vi "Util_Trajectory_WriteFile_Config.vi"(9 "TRAJECTORY_CONFIG":T1 {"End Velocity" format="%20.4f"; "StartVelocity" format="%20.4f"; "Max Acceleration" format="%20.4f"; "MaxVelocity" format="%20.4f"}, 11 "Byte Steam File In":refnum<file>) -> (0 "error out":errorcluster, 3 "Byte Steam File Out":refnum<file>)   [LabVIEW 2019, in "Trajectory_Library.lvlib"]
doc: "Internal routine to write the Trajectory Configuration data to a file.\n\nParameters:\n - ByteStream In - File stream\n - TrajectoryConfig - Data structure containing trajectory configuration\n\nReturns:\n - ByteStream Out - File stream\n - Error out - returned error cluster\n\nReturns:\n - outTrajectory - Trajectory data structure\n - Error out - returned error cluster"
uses:
  Trajectory_Library.lvlib
  TypeDef/TRAJ_CONFIG.ctl
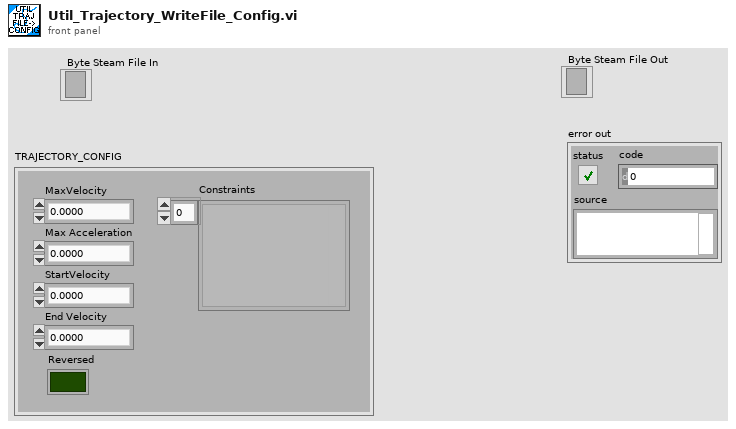
[diagram p1: front panel]
types:
  T1 = typedef "Trajectory_Library.lvlib/TRAJ_CONFIG.ctl" = cluster{"MaxVelocity":dbl, "Max Acceleration":dbl, "StartVelocity":dbl, "End Velocity":dbl, "Reversed":bool, "Constraints":variant[]}
  T2 = typedef "WPILib_Math.lvlib/TRAJ_CONSTRAINT_DIIF_DRIVE_KINEMATICS.ctl" = cluster{"Max Speed (M/S)":dbl, "DIFF_DRIVE_KINEMATICS":T3, "Max Accel (M/S2)":dbl}
  T3 = typedef "WPILib_Math.lvlib/DIFF_DRIVE_KINEMATICS.ctl" = cluster{"TrackWidth_Meters":dbl}
  T4 = typedef "Trajectory_Library.lvlib/TRAJ_CONSTRAINT_DIIF_DRIVE_VOLTAGE.ctl" = cluster{"Max Voltage":dbl, "DIFF_DRIVE_KINEMATICS":T5, "SIMPLE_MOTOR_FF":T6}
  T5 = typedef "Trajectory_Library.lvlib/DIFF_DRIVE_KINEMATICS.ctl" = cluster{"TrackWidth_Meters":dbl}
  T6 = typedef "Trajectory_Library.lvlib/SIMPLE_MOTOR_FF.ctl" = cluster{"Ks":dbl, "Kv":dbl, "Ka":dbl, "KnInv":dbl}
  T7 = typedef "Trajectory_Library.lvlib/TRAJ_CONSTRAINT_SWERVE_DRIVE_KINEMATICS.ctl" = cluster{"Max Speed (M/S)":dbl, "SwerveKinematics":T8}
  T8 = typedef "Trajectory_Library.lvlib/SWERVE_DRIVE_KINEMATICS.ctl" = cluster{"NumModules":i32, "InverseKinematics":T9, "ForwardKinematics":T9, "Modules":T10[], "PrevCoR":T10, "SavedModuleStates":T11[]}
  T9 = typedef "NI_Matrix.lvlib/RealMatrix.ctl" = dbl[][]
  T10 = typedef "Trajectory_Library.lvlib/TRANSLATION2D.ctl" = cluster{"X":dbl, "Y":dbl}
  T11 = typedef "Trajectory_Library.lvlib/SWERVE_DRIVE_MODULE_STATE.ctl" = cluster{"Speed":dbl, "Angle":T12}
  T12 = typedef "Trajectory_Library.lvlib/ROTATION2D.ctl" = cluster{"VALUE":dbl, "COS":dbl, "SIN":dbl}
  T13 = typedef "Trajectory_Library.lvlib/TRAJ_CONSTRAINT_MECA_DRIVE_KINEMATICS.ctl" = cluster{"Max Speed (M/S)":dbl, "MECA_DRIVE_KINEMATICS":T14}
  T14 = typedef "Trajectory_Library.lvlib/MECA_DRIVE_KINEMATICS.ctl" = cluster{"FrontLeft":T10, "FrontRight":T10, "RearLeft":T10, "RearRight":T10, "InverseKinematics":T9, "ForwardKinematics":T9, "PrevCoR":T10}
  T15 = typedef "Trajectory_Library.lvlib/TRAJ_CONSTRAINT_CENTRIPETAL_ACCEL.ctl" = cluster{"Max Cent Accel":dbl}
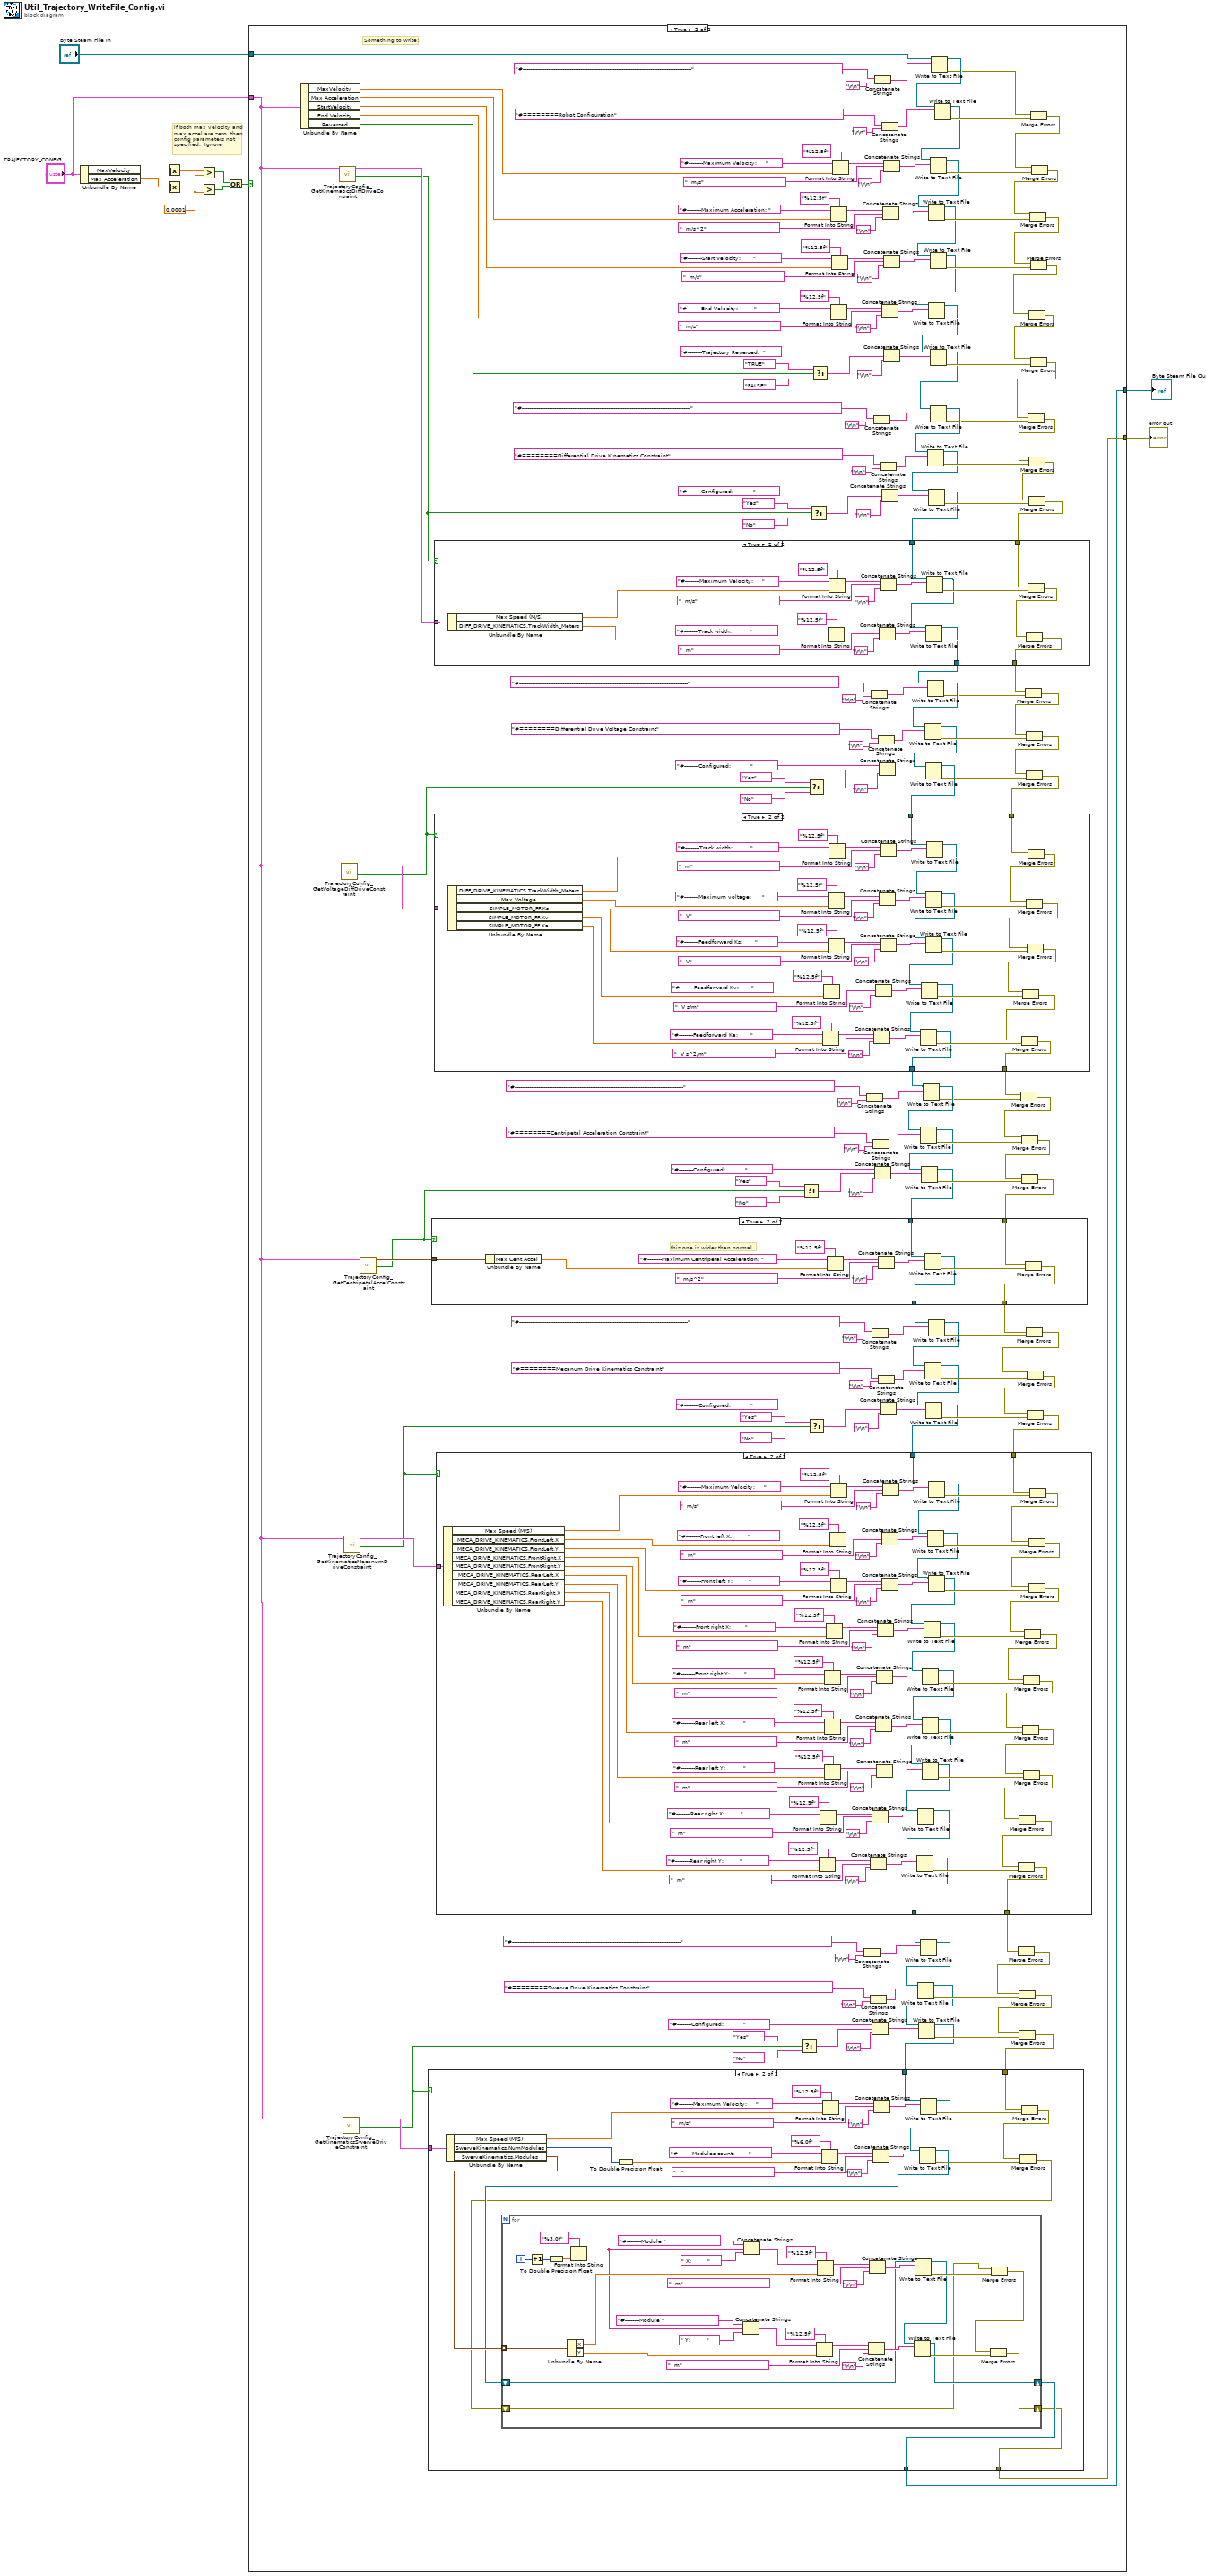
[diagram p0: block diagram]
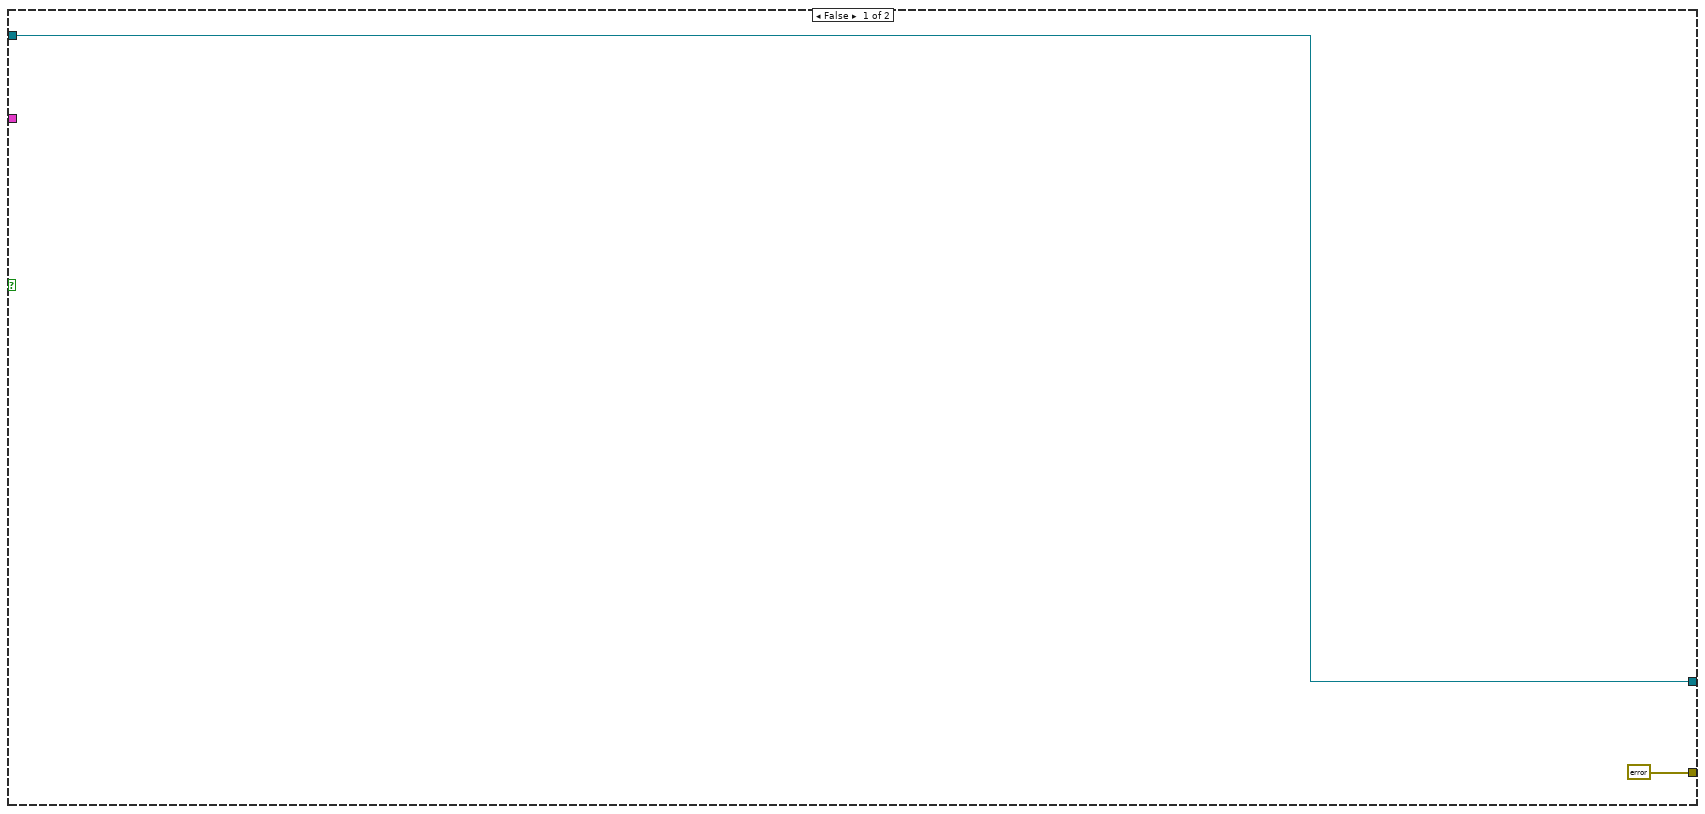
[diagram p2: hidden frame]
diagram:
  w5 = 0.0001
  # "if both max velocity and\nmax accel are zero, then\nconfig parameters not\nspecified.  Ignore"
  n1 = Unbundle By Name("TRAJECTORY_CONFIG") -> ("MaxVelocity"=w8:dbl, "Max Acceleration"=w9:dbl)
  n2 = Absolute Value(x=w8) -> (abs(x)=w7:dbl)
  n3 = Absolute Value(x=w9) -> (abs(x)=w6:dbl)
  n4 = Greater?(x=w7, y=w5) -> (0:w4:bool)
  n5 = Greater?(x=w6, y=w5) -> (0:w3:bool)
  n6 = Or(x=w4, y=w3) -> (x .or. y?=w2:bool)
  n7 = case shown="True" w2 {
    tunnel: [w14 w26] -> w12
    tunnel: "Byte Steam File In" -> [w14 w196]
    tunnel: [errorcluster {"status"=FALSE, "code"=0, "source"=""} ("error out") w27] -> w10
    tunnel: "TRAJECTORY_CONFIG" -> [_ w15]
    frame False {
    }
    frame True {
      # "Something to write!"
      n8 = Unbundle By Name(w15) -> ("MaxVelocity"=w182:dbl, "Max Acceleration"=w181:dbl, "StartVelocity"=w163:dbl, "End Velocity"=w162:dbl, "Reversed"=w161:bool)
      n9 = call "TrajectoryConfig_GetKinematicsDiffDriveContraint.vi"("inTRAJECTORY_CONFIG"=w15) -> ("Constraint Exists"=w24:bool, "Diff Drive Kinematics Constraint"=w25:T2)  [unwired: 9 in]
      n10 = call "TrajectoryConfig_GetVoltageDiffDriveConstraint.vi"("inTRAJECTORY_CONFIG"=w15) -> ("Constraint Exists"=w22:bool, "Differential Drive Voltage Constraint"=w23:T4)  [unwired: 9 in]
      n11 = call "TrajectoryConfig_GetKinematicsSwerveDriveConstraint.vi"("inTRAJECTORY_CONFIG"=w15) -> ("Constraint Exists"=w16:bool, "Swerver Drive Kinematics Constraint"=w19:T7)  [unwired: 9 in]
      n12 = call "TrajectoryConfig_GetKinematicsMecanumDriveConstraint.vi"("inTRAJECTORY_CONFIG"=w15) -> ("Constraint Exists"=w17:bool, "Mecanum Drive Kinematics Constraint"=w18:T13)  [unwired: 9 in]
      n13 = call "TrajectoryConfig_GetCentripetalAccelConstraint.vi"("inTRAJECTORY_CONFIG"=w15) -> ("Constraint Exists"=w20:bool, "Centripital Accleration Constraint"=w21:T15)  [unwired: 9 in]
      n14 = Select(t="Yes" ("string"), s=w16, f="No" ("string")) -> (s? t:f=w79:string)
      n15 = Select(t="Yes" ("string"), s=w20, f="No" ("string")) -> (s? t:f=w111:string)
      n16 = Select(t="Yes" ("string"), s=w22, f="No" ("string")) -> (s? t:f=w127:string)
      n17 = Select(t="Yes" ("string"), s=w17, f="No" ("string")) -> (s? t:f=w95:string)
      n18 = Select(t="Yes" ("string"), s=w24, f="No" ("string")) -> (s? t:f=w151:string)
      n19 = Select(t="TRUE" ("string"), s=w161, f="FALSE" ("string")) -> (s? t:f=w167:string)
      n20 = Format Into String(format string="%12.5f", initial string="#--------End Velocity:         " ("string"), w162) -> (resulting string=w171:string)  [unwired: 1 in, 1 out]
      n21 = Format Into String(format string="%12.5f", initial string="#--------Maximum Acceleration: " ("string"), w181) -> (resulting string=w183:string)  [unwired: 1 in, 1 out]
      n22 = Format Into String(format string="%12.5f", initial string="#--------Start Velocity:       " ("string"), w163) -> (resulting string=w176:string)  [unwired: 1 in, 1 out]
      n23 = Format Into String(format string="%12.5f", initial string="#--------Maximum Velocity:     " ("string"), w182) -> (resulting string=w188:string)  [unwired: 1 in, 1 out]
      n24 = Concatenate Strings("#----------------------------------------------------------------------------------------------" ("string"), "\r\n") -> (w83:string)
      n25 = Concatenate Strings("#----------------------------------------------------------------------------------------------" ("string"), "\r\n") -> (w115:string)
      n26 = Concatenate Strings("#========Swerve Drive Kinematics Constraint" ("string"), "\r\n") -> (w86:string)
      n27 = Concatenate Strings("#----------------------------------------------------------------------------------------------" ("string"), "\r\n") -> (w131:string)
      n28 = Concatenate Strings("#----------------------------------------------------------------------------------------------" ("string"), "\r\n") -> (w99:string)
      n29 = Concatenate Strings("#--------Configured:           " ("string"), w79, "\r\n") -> (w81:string)
      n30 = Concatenate Strings("#========Centripetal Acceleration Constraint" ("string"), "\r\n") -> (w118:string)
      n31 = Concatenate Strings("#----------------------------------------------------------------------------------------------" ("string"), "\r\n") -> (w155:string)
      n32 = Concatenate Strings("#----------------------------------------------------------------------------------------------" ("string"), "\r\n") -> (w197:string)
      n33 = Concatenate Strings("#--------Configured:           " ("string"), w111, "\r\n") -> (w113:string)
      n34 = Concatenate Strings("#========Differential Drive Voltage Constraint" ("string"), "\r\n") -> (w134:string)
      n35 = Concatenate Strings("#========Mecanum Drive Kinematics Constraint" ("string"), "\r\n") -> (w102:string)
      n36 = Concatenate Strings("#--------Configured:           " ("string"), w127, "\r\n") -> (w129:string)
      n37 = Concatenate Strings("#--------Configured:           " ("string"), w95, "\r\n") -> (w97:string)
      n38 = Concatenate Strings("#========Differential Drive Kinematics Constraint" ("string"), "\r\n") -> (w158:string)
      n39 = Concatenate Strings("#========Robot Configuration" ("string"), "\r\n") -> (w200:string)
      n40 = Concatenate Strings(w171, "  m/s" ("string"), "\r\n") -> (w173:string)
      n41 = Concatenate Strings("#--------Configured:           " ("string"), w151, "\r\n") -> (w153:string)
      n42 = Concatenate Strings(w183, "  m/s^2" ("string"), "\r\n") -> (w185:string)
      n43 = Concatenate Strings(w176, "  m/s" ("string"), "\r\n") -> (w178:string)
      n44 = Concatenate Strings("#--------Trajectory Reversed:  " ("string"), w167, "\r\n") -> (w169:string)
      n45 = Concatenate Strings(w188, "  m/s" ("string"), "\r\n") -> (w192:string)
      n46 = Write to Text File(file (use dialog)=w196, text=w197) -> (refnum out=w195:refnum<file>, error out=w189:errorcluster)  [unwired: 2 in, 1 out]
      n47 = Write to Text File(file (use dialog)=w195, text=w200) -> (refnum out=w72:refnum<file>, error out=w191:errorcluster)  [unwired: 2 in, 1 out]
      n48 = Write to Text File(file (use dialog)=w72, text=w192) -> (refnum out=w71:refnum<file>, error out=w190:errorcluster)  [unwired: 2 in, 1 out]
      n49 = Write to Text File(file (use dialog)=w71, text=w185) -> (refnum out=w70:refnum<file>, error out=w184:errorcluster)  [unwired: 2 in, 1 out]
      n50 = Write to Text File(file (use dialog)=w70, text=w178) -> (refnum out=w69:refnum<file>, error out=w177:errorcluster)  [unwired: 2 in, 1 out]
      n51 = Write to Text File(file (use dialog)=w69, text=w173) -> (refnum out=w68:refnum<file>, error out=w172:errorcluster)  [unwired: 2 in, 1 out]
      n52 = Write to Text File(file (use dialog)=w68, text=w169) -> (refnum out=w67:refnum<file>, error out=w168:errorcluster)  [unwired: 2 in, 1 out]
      n53 = Write to Text File(file (use dialog)=w67, text=w155) -> (refnum out=w147:refnum<file>, error out=w137:errorcluster)  [unwired: 2 in, 1 out]
      n54 = Write to Text File(file (use dialog)=w147, text=w158) -> (refnum out=w66:refnum<file>, error out=w138:errorcluster)  [unwired: 2 in, 1 out]
      n55 = Write to Text File(file (use dialog)=w66, text=w153) -> (refnum out=w65:refnum<file>, error out=w152:errorcluster)  [unwired: 2 in, 1 out]
      n56 = Merge Errors(w189, w191) -> (w55:errorcluster)
      n57 = Merge Errors(w55, w190) -> (w54:errorcluster)
      n58 = Merge Errors(w54, w184) -> (w53:errorcluster)
      n59 = Merge Errors(w53, w177) -> (w52:errorcluster)
      n60 = Merge Errors(w52, w172) -> (w51:errorcluster)
      n61 = Merge Errors(w51, w168) -> (w50:errorcluster)
      n62 = Merge Errors(w50, w137) -> (w49:errorcluster)
      n63 = Merge Errors(w49, w138) -> (w48:errorcluster)
      n64 = Merge Errors(w48, w152) -> (w47:errorcluster)
      n65 = case shown="True" w24 {
        tunnel: w25 -> [_ w453]
        tunnel: w65 -> [w430 w436]
        tunnel: [w430 w434] -> w64
        tunnel: w47 -> [w429 w433]
        tunnel: [w429 w431] -> w46
        frame False {
        }
        frame True {
          n66 = Unbundle By Name(w453) -> ("Max Speed (M/S)"=w442:dbl, "DIFF_DRIVE_KINEMATICS.TrackWidth_Meters"=w441:dbl)
          n67 = Format Into String(format string="%12.5f", initial string="#--------Track width:          " ("string"), w441) -> (resulting string=w443:string)  [unwired: 1 in, 1 out]
          n68 = Format Into String(format string="%12.5f", initial string="#--------Maximum Velocity:     " ("string"), w442) -> (resulting string=w448:string)  [unwired: 1 in, 1 out]
          n69 = Concatenate Strings(w443, "  m" ("string"), "\r\n") -> (w445:string)
          n70 = Concatenate Strings(w448, "  m/s" ("string"), "\r\n") -> (w450:string)
          n71 = Write to Text File(file (use dialog)=w436, text=w450) -> (refnum out=w435:refnum<file>, error out=w449:errorcluster)  [unwired: 2 in, 1 out]
          n72 = Write to Text File(file (use dialog)=w435, text=w445) -> (refnum out=w434:refnum<file>, error out=w444:errorcluster)  [unwired: 2 in, 1 out]
          n73 = Merge Errors(w433, w449) -> (w432:errorcluster)
          n74 = Merge Errors(w432, w444) -> (w431:errorcluster)
        }
      }
      n75 = Write to Text File(file (use dialog)=w64, text=w131) -> (refnum out=w123:refnum<file>, error out=w121:errorcluster)  [unwired: 2 in, 1 out]
      n76 = Write to Text File(file (use dialog)=w123, text=w134) -> (refnum out=w63:refnum<file>, error out=w122:errorcluster)  [unwired: 2 in, 1 out]
      n77 = Write to Text File(file (use dialog)=w63, text=w129) -> (refnum out=w62:refnum<file>, error out=w128:errorcluster)  [unwired: 2 in, 1 out]
      n78 = Merge Errors(w46, w121) -> (w45:errorcluster)
      n79 = Merge Errors(w45, w122) -> (w44:errorcluster)
      n80 = Merge Errors(w44, w128) -> (w43:errorcluster)
      n81 = case shown="True" w22 {
        tunnel: w23 -> [_ w428]
        tunnel: w62 -> [w375 w387]
        tunnel: [w375 w382] -> w61
        tunnel: w43 -> [w374 w381]
        tunnel: [w374 w376] -> w42
        frame False {
        }
        frame True {
          n82 = Unbundle By Name(w428) -> ("DIFF_DRIVE_KINEMATICS.TrackWidth_Meters"=w417:dbl, "Max Voltage"=w416:dbl, "SIMPLE_MOTOR_FF.Ks"=w390:dbl, "SIMPLE_MOTOR_FF.Kv"=w389:dbl, "SIMPLE_MOTOR_FF.Ka"=w388:dbl)
          n83 = Format Into String(format string="%12.5f", initial string="#--------Feedforward Ka:       " ("string"), w388) -> (resulting string=w393:string)  [unwired: 1 in, 1 out]
          n84 = Format Into String(format string="%12.5f", initial string="#--------Feedforward Kv:       " ("string"), w389) -> (resulting string=w400:string)  [unwired: 1 in, 1 out]
          n85 = Format Into String(format string="%12.5f", initial string="#--------Maximum voltage:      " ("string"), w416) -> (resulting string=w418:string)  [unwired: 1 in, 1 out]
          n86 = Format Into String(format string="%12.5f", initial string="#--------Feedforward Ks:       " ("string"), w390) -> (resulting string=w407:string)  [unwired: 1 in, 1 out]
          n87 = Format Into String(format string="%12.5f", initial string="#--------Track width:          " ("string"), w417) -> (resulting string=w423:string)  [unwired: 1 in, 1 out]
          n88 = Concatenate Strings(w393, "  V s^2/m" ("string"), "\r\n") -> (w395:string)
          n89 = Concatenate Strings(w400, "  V s/m" ("string"), "\r\n") -> (w402:string)
          n90 = Concatenate Strings(w418, "  V" ("string"), "\r\n") -> (w420:string)
          n91 = Concatenate Strings(w407, "  V" ("string"), "\r\n") -> (w409:string)
          n92 = Concatenate Strings(w423, "  m" ("string"), "\r\n") -> (w425:string)
          n93 = Write to Text File(file (use dialog)=w387, text=w425) -> (refnum out=w386:refnum<file>, error out=w424:errorcluster)  [unwired: 2 in, 1 out]
          n94 = Write to Text File(file (use dialog)=w386, text=w420) -> (refnum out=w385:refnum<file>, error out=w419:errorcluster)  [unwired: 2 in, 1 out]
          n95 = Write to Text File(file (use dialog)=w385, text=w409) -> (refnum out=w384:refnum<file>, error out=w408:errorcluster)  [unwired: 2 in, 1 out]
          n96 = Write to Text File(file (use dialog)=w384, text=w402) -> (refnum out=w383:refnum<file>, error out=w401:errorcluster)  [unwired: 2 in, 1 out]
          n97 = Write to Text File(file (use dialog)=w383, text=w395) -> (refnum out=w382:refnum<file>, error out=w394:errorcluster)  [unwired: 2 in, 1 out]
          n98 = Merge Errors(w381, w424) -> (w380:errorcluster)
          n99 = Merge Errors(w380, w419) -> (w379:errorcluster)
          n100 = Merge Errors(w379, w408) -> (w378:errorcluster)
          n101 = Merge Errors(w378, w401) -> (w377:errorcluster)
          n102 = Merge Errors(w377, w394) -> (w376:errorcluster)
        }
      }
      n103 = Write to Text File(file (use dialog)=w61, text=w115) -> (refnum out=w107:refnum<file>, error out=w105:errorcluster)  [unwired: 2 in, 1 out]
      n104 = Write to Text File(file (use dialog)=w107, text=w118) -> (refnum out=w60:refnum<file>, error out=w106:errorcluster)  [unwired: 2 in, 1 out]
      n105 = Write to Text File(file (use dialog)=w60, text=w113) -> (refnum out=w59:refnum<file>, error out=w112:errorcluster)  [unwired: 2 in, 1 out]
      n106 = Merge Errors(w42, w105) -> (w41:errorcluster)
      n107 = Merge Errors(w41, w106) -> (w40:errorcluster)
      n108 = Merge Errors(w40, w112) -> (w39:errorcluster)
      n109 = case shown="True" w20 {
        tunnel: w21 -> [_ w373]
        tunnel: w59 -> [w360 w364]
        tunnel: [w360 w363] -> w58
        tunnel: w39 -> [w359 w362]
        tunnel: [w359 w361] -> w38
        frame False {
        }
        frame True {
          # "this one is wider than normal..."
          n110 = Unbundle By Name(w373) -> ("Max Cent Accel"=w367:dbl)
          n111 = Format Into String(format string="%12.5f", initial string="#--------Maximum Centripetal Acceleration: " ("string"), w367) -> (resulting string=w368:string)  [unwired: 1 in, 1 out]
          n112 = Concatenate Strings(w368, "  m/s^2" ("string"), "\r\n") -> (w370:string)
          n113 = Write to Text File(file (use dialog)=w364, text=w370) -> (refnum out=w363:refnum<file>, error out=w369:errorcluster)  [unwired: 2 in, 1 out]
          n114 = Merge Errors(w362, w369) -> (w361:errorcluster)
        }
      }
      n115 = Write to Text File(file (use dialog)=w58, text=w99) -> (refnum out=w91:refnum<file>, error out=w89:errorcluster)  [unwired: 2 in, 1 out]
      n116 = Write to Text File(file (use dialog)=w91, text=w102) -> (refnum out=w57:refnum<file>, error out=w90:errorcluster)  [unwired: 2 in, 1 out]
      n117 = Write to Text File(file (use dialog)=w57, text=w97) -> (refnum out=w33:refnum<file>, error out=w96:errorcluster)  [unwired: 2 in, 1 out]
      n118 = Merge Errors(w38, w89) -> (w37:errorcluster)
      n119 = Merge Errors(w37, w90) -> (w36:errorcluster)
      n120 = Merge Errors(w36, w96) -> (w32:errorcluster)
      n121 = case shown="True" w17 {
        tunnel: w18 -> [_ w358]
        tunnel: w33 -> [w265 w320]
        tunnel: [w265 w267] -> w31
        tunnel: w32 -> [w264 w315]
        tunnel: [w264 w266] -> w30
        frame False {
        }
        frame True {
          n122 = Unbundle By Name(w358) -> ("Max Speed (M/S)"=w347:dbl, "MECA_DRIVE_KINEMATICS.FrontLeft.X"=w346:dbl, "MECA_DRIVE_KINEMATICS.FrontLeft.Y"=w308:dbl, "MECA_DRIVE_KINEMATICS.FrontRight.X"=w310:dbl, "MECA_DRIVE_KINEMATICS.FrontRight.Y"=w309:dbl, "MECA_DRIVE_KINEMATICS.RearLeft.X"=w271:dbl, "MECA_DRIVE_KINEMATICS.RearLeft.Y"=w270:dbl, "MECA_DRIVE_KINEMATICS.RearRight.X"=w269:dbl, "MECA_DRIVE_KINEMATICS.RearRight.Y"=w268:dbl)
          n123 = Format Into String(format string="%12.5f", initial string="#--------Rear right Y:         " ("string"), w268) -> (resulting string=w282:string)  [unwired: 1 in, 1 out]
          n124 = Format Into String(format string="%12.5f", initial string="#--------Rear right X:         " ("string"), w269) -> (resulting string=w289:string)  [unwired: 1 in, 1 out]
          n125 = Format Into String(format string="%12.5f", initial string="#--------Rear left X:          " ("string"), w271) -> (resulting string=w303:string)  [unwired: 1 in, 1 out]
          n126 = Format Into String(format string="%12.5f", initial string="#--------Front right Y:        " ("string"), w309) -> (resulting string=w323:string)  [unwired: 1 in, 1 out]
          n127 = Format Into String(format string="%12.5f", initial string="#--------Rear left Y:          " ("string"), w270) -> (resulting string=w296:string)  [unwired: 1 in, 1 out]
          n128 = Format Into String(format string="%12.5f", initial string="#--------Front right X:        " ("string"), w310) -> (resulting string=w330:string)  [unwired: 1 in, 1 out]
          n129 = Format Into String(format string="%12.5f", initial string="#--------Front left X:         " ("string"), w346) -> (resulting string=w348:string)  [unwired: 1 in, 1 out]
          n130 = Format Into String(format string="%12.5f", initial string="#--------Front left Y:         " ("string"), w308) -> (resulting string=w337:string)  [unwired: 1 in, 1 out]
          n131 = Format Into String(format string="%12.5f", initial string="#--------Maximum Velocity:     " ("string"), w347) -> (resulting string=w353:string)  [unwired: 1 in, 1 out]
          n132 = Concatenate Strings(w282, "  m" ("string"), "\r\n") -> (w284:string)
          n133 = Concatenate Strings(w289, "  m" ("string"), "\r\n") -> (w291:string)
          n134 = Concatenate Strings(w303, "  m" ("string"), "\r\n") -> (w305:string)
          n135 = Concatenate Strings(w323, "  m" ("string"), "\r\n") -> (w325:string)
          n136 = Concatenate Strings(w296, "  m" ("string"), "\r\n") -> (w298:string)
          n137 = Concatenate Strings(w330, "  m" ("string"), "\r\n") -> (w332:string)
          n138 = Concatenate Strings(w348, "  m" ("string"), "\r\n") -> (w350:string)
          n139 = Concatenate Strings(w337, "  m" ("string"), "\r\n") -> (w339:string)
          n140 = Concatenate Strings(w353, "  m/s" ("string"), "\r\n") -> (w355:string)
          n141 = Write to Text File(file (use dialog)=w320, text=w355) -> (refnum out=w319:refnum<file>, error out=w354:errorcluster)  [unwired: 2 in, 1 out]
          n142 = Write to Text File(file (use dialog)=w319, text=w350) -> (refnum out=w318:refnum<file>, error out=w349:errorcluster)  [unwired: 2 in, 1 out]
          n143 = Write to Text File(file (use dialog)=w318, text=w339) -> (refnum out=w317:refnum<file>, error out=w338:errorcluster)  [unwired: 2 in, 1 out]
          n144 = Write to Text File(file (use dialog)=w317, text=w332) -> (refnum out=w316:refnum<file>, error out=w331:errorcluster)  [unwired: 2 in, 1 out]
          n145 = Write to Text File(file (use dialog)=w316, text=w325) -> (refnum out=w273:refnum<file>, error out=w324:errorcluster)  [unwired: 2 in, 1 out]
          n146 = Write to Text File(file (use dialog)=w273, text=w305) -> (refnum out=w279:refnum<file>, error out=w304:errorcluster)  [unwired: 2 in, 1 out]
          n147 = Write to Text File(file (use dialog)=w279, text=w298) -> (refnum out=w278:refnum<file>, error out=w297:errorcluster)  [unwired: 2 in, 1 out]
          n148 = Write to Text File(file (use dialog)=w278, text=w291) -> (refnum out=w277:refnum<file>, error out=w290:errorcluster)  [unwired: 2 in, 1 out]
          n149 = Write to Text File(file (use dialog)=w277, text=w284) -> (refnum out=w267:refnum<file>, error out=w283:errorcluster)  [unwired: 2 in, 1 out]
          n150 = Merge Errors(w315, w354) -> (w314:errorcluster)
          n151 = Merge Errors(w314, w349) -> (w313:errorcluster)
          n152 = Merge Errors(w313, w338) -> (w312:errorcluster)
          n153 = Merge Errors(w312, w331) -> (w311:errorcluster)
          n154 = Merge Errors(w311, w324) -> (w272:errorcluster)
          n155 = Merge Errors(w272, w304) -> (w276:errorcluster)
          n156 = Merge Errors(w276, w297) -> (w275:errorcluster)
          n157 = Merge Errors(w275, w290) -> (w274:errorcluster)
          n158 = Merge Errors(w274, w283) -> (w266:errorcluster)
        }
      }
      n159 = Write to Text File(file (use dialog)=w31, text=w83) -> (refnum out=w75:refnum<file>, error out=w73:errorcluster)  [unwired: 2 in, 1 out]
      n160 = Write to Text File(file (use dialog)=w75, text=w86) -> (refnum out=w56:refnum<file>, error out=w74:errorcluster)  [unwired: 2 in, 1 out]
      n161 = Write to Text File(file (use dialog)=w56, text=w81) -> (refnum out=w28:refnum<file>, error out=w80:errorcluster)  [unwired: 2 in, 1 out]
      n162 = Merge Errors(w30, w73) -> (w35:errorcluster)
      n163 = Merge Errors(w35, w74) -> (w34:errorcluster)
      n164 = Merge Errors(w34, w80) -> (w29:errorcluster)
      n165 = case shown="True" w16 {
        tunnel: w19 -> [_ w231]
        tunnel: w28 -> [w204 w215]
        tunnel: [w204 w206] -> w26
        tunnel: w29 -> [w203 w213]
        tunnel: [w203 w205] -> w27
        frame False {
        }
        frame True {
          n166 = Unbundle By Name(w231) -> ("Max Speed (M/S)"=w220:dbl, "SwerveKinematics.NumModules"=w211:i32, "SwerveKinematics.Modules"=w209:T10[])
          n167 = To Double Precision Float(number=w211) -> (double precision float=w210:dbl)
          n168 = Format Into String(format string="%6.0f", initial string="#--------Modules count:        " ("string"), w210) -> (resulting string=w221:string)  [unwired: 1 in, 1 out]
          n169 = Format Into String(format string="%12.5f", initial string="#--------Maximum Velocity:     " ("string"), w220) -> (resulting string=w226:string)  [unwired: 1 in, 1 out]
          n170 = Concatenate Strings(w221, "   " ("string"), "\r\n") -> (w223:string)
          n171 = Concatenate Strings(w226, "  m/s" ("string"), "\r\n") -> (w228:string)
          n172 = Write to Text File(file (use dialog)=w215, text=w228) -> (refnum out=w214:refnum<file>, error out=w227:errorcluster)  [unwired: 2 in, 1 out]
          n173 = Write to Text File(file (use dialog)=w214, text=w223) -> (refnum out=w208:refnum<file>, error out=w222:errorcluster)  [unwired: 2 in, 1 out]
          n174 = Merge Errors(w213, w227) -> (w212:errorcluster)
          n175 = Merge Errors(w212, w222) -> (w207:errorcluster)
          n176 = for {
            tunnel: w209 -> [w249] mode=indexing
            shift-right: [w235] -> w206
            shift-left: w208 -> [w233]
            shift-right: [w234] -> w205
            shift-left: w207 -> [w232]
            i -> [w247]
            n177 = Increment(x=w247) -> (x+1=w246:i32)
            n178 = To Double Precision Float(number=w246) -> (double precision float=w245:dbl)
            n179 = Unbundle By Name(w249) -> ("X"=w241:dbl, "Y"=w236:dbl)
            n180 = Format Into String(format string="%3.0f", w245) -> (resulting string=w237:string)  [unwired: 2 in, 1 out]
            n181 = Concatenate Strings("#--------Module " ("string"), w237, " Y:         " ("string")) -> (w238:string)
            n182 = Concatenate Strings("#--------Module " ("string"), w237, " X:         " ("string")) -> (w242:string)
            n183 = Format Into String(format string="%12.5f", initial string=w238, w236) -> (resulting string=w254:string)  [unwired: 1 in, 1 out]
            n184 = Format Into String(format string="%12.5f", initial string=w242, w241) -> (resulting string=w260:string)  [unwired: 1 in, 1 out]
            n185 = Concatenate Strings(w254, "  m" ("string"), "\r\n") -> (w256:string)
            n186 = Concatenate Strings(w260, "  m" ("string"), "\r\n") -> (w262:string)
            n187 = Write to Text File(file (use dialog)=w233, text=w262) -> (refnum out=w251:refnum<file>, error out=w261:errorcluster)  [unwired: 2 in, 1 out]
            n188 = Write to Text File(file (use dialog)=w251, text=w256) -> (refnum out=w235:refnum<file>, error out=w255:errorcluster)  [unwired: 2 in, 1 out]
            n189 = Merge Errors(w232, w261) -> (w250:errorcluster)
            n190 = Merge Errors(w250, w255) -> (w234:errorcluster)
          }
        }
      }
    }
  }
  "error out" <- w10
  "Byte Steam File Out" <- w12
